vi "Draw.vi"(8 "error in (no error)":errorcluster, 10 "2D Picture in":picture, 11 "Point in":refnum<class "PointSpecialized.lvclass">) -> (0 "error out":errorcluster, 2 "2D Picture out":picture, 3 "Point out":refnum<class "PointSpecialized.lvclass">)   [LabVIEW 2021, in "Picture2D.lvlib" / "PointSpecialized.lvclass"]
uses:
  PointSpecialized.lvclass
  PointSpecialized.lvclass/PointSpecialized.ctl
  Color/Color.lvclass
  Pen/Pen.lvclass
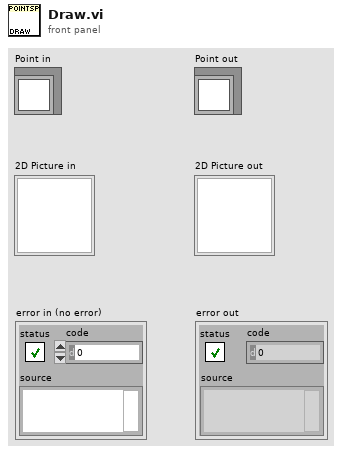
[diagram p1: front panel]
types:
  T1 = cluster{"Width":u16, "Style":enum32{"Solid", "Dash", "Dot", "DashDot", "DashDotDot"}}
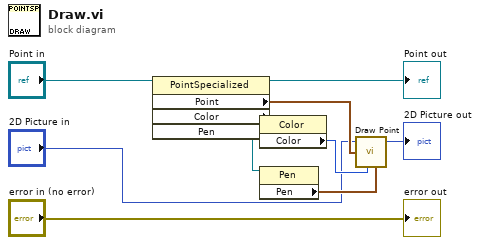
[diagram p0: block diagram]
diagram:
  n1 = property class="PointSpecialized"(reference="Point in") -> (reference out=→"Point out":refnum<class "PointSpecialized.lvclass">, "Point"=w8:cluster{"x":i16, "y":i16}, "Color"=w7:refnum<class "Color.lvclass">, "Pen"=w5:refnum<class "Pen.lvclass">)  [unwired: 1 in, 1 out]
  n2 = property class="Color"(reference=w7) -> ("Color"=w6:u32)  [unwired: 1 in, 2 out]
  n3 = property class="Pen"(reference=w5) -> ("Pen"=w4:T1)  [unwired: 1 in, 2 out]
  n4 = call <vilib>:"Draw Point.vi"("picture"="2D Picture in", "point(x,y)"=w8, "color(black)"=w6, "pen"=w4) -> ("new picture"=→"2D Picture out":picture)  [unwired: 5 in]
  "error out" <- "error in (no error)"
